vi "Ej 21 Solid.vi"() -> ()   [LabVIEW 2020]
uses:
  <vilib>/Motion/Express/_s/nimc.ex.straightLineMove.startStraightLineMove.axis.modeAbsolute.0.vi
  <vilib>/Motion/BlockNode/FB.NIMotion.xnode
panel:
  in  "position":dbl=1000.0
  in  "stop":bool
  # "Controlador para la posición del mecanismo"
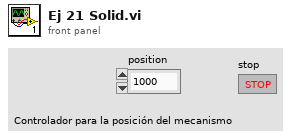
[diagram p1: front panel]
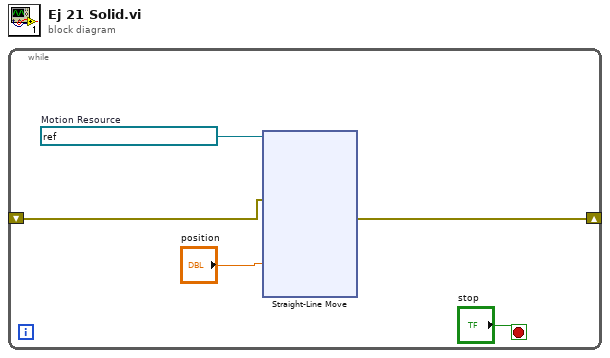
[diagram p0: block diagram]
diagram:
  n1 = while {
    shift-right: [w3] -> _
    shift-left: _ -> [w2]
    stop <- "stop" stop-if-true
    w4 = refnum<k21> "nism://My Computer/Axis 1"  # Motion Resource
    n2 = xnode ("Straight-Line Move")("position"="position", "resource"=w4, "error in"=w2) -> ("error out"=w3:errorcluster)  [unwired: 7 in, 2 out]
  }
